vi "OP600ZP_FDT_FIN.vi"(8 "errin":errorcluster) -> (0 "errout":errorcluster caption="sortie d'erreur", 1 "ToBDD":T1, 2 "Log":string, 3 "is OK?":bool)   [LabVIEW 2020]
uses:
  OP600ZP_VGConf.vi
  VG/IS30%.vi
panel:
  out "PASS/FAIL?":string
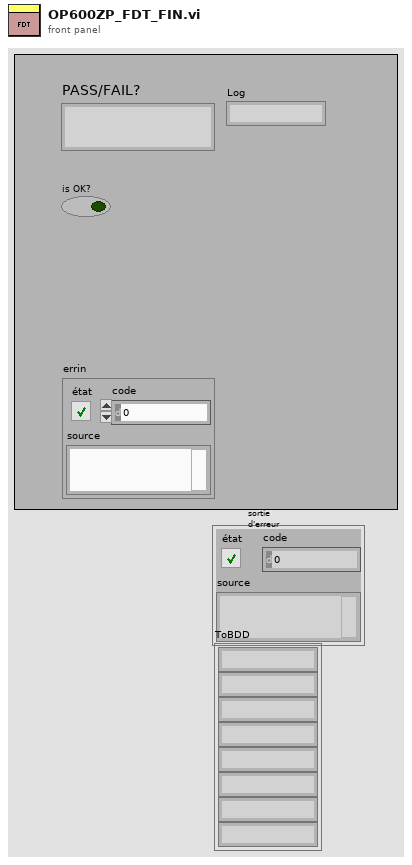
[diagram p1: front panel]
types:
  T1 = cluster{string, string, string, string, string, string, string, string}
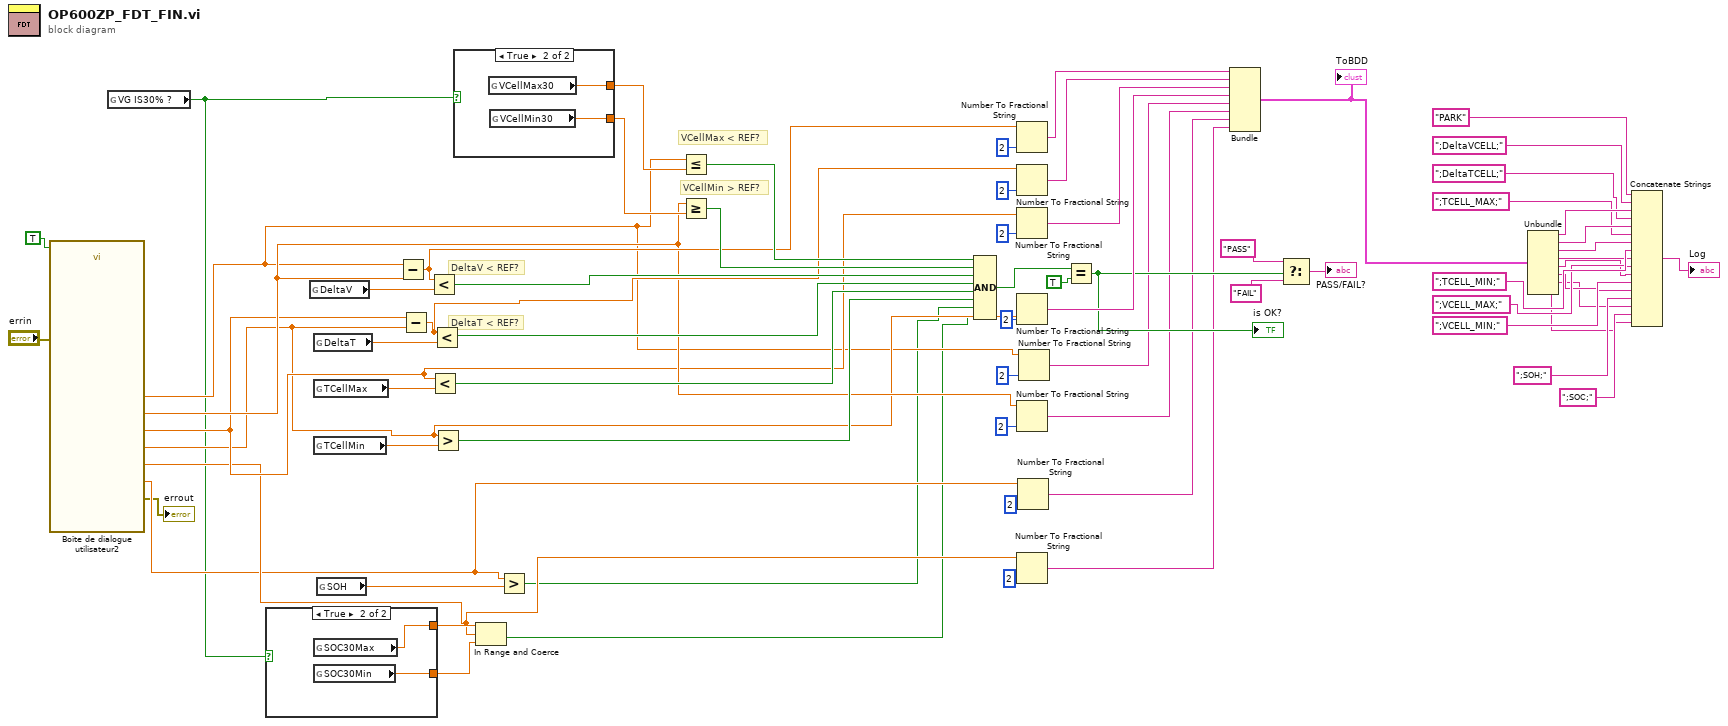
[diagram p0: block diagram]
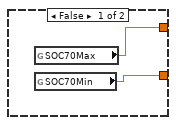
[diagram p2: hidden frame]
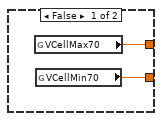
[diagram p3: hidden frame]
diagram:
  # "DeltaT < REF?"
  # "DeltaV < REF?"
  # "VCellMin > REF?"
  # "VCellMax < REF?"
  n1 = call "Boîte de dialogue utilisateur2"("Enable"=TRUE, "error in (no error)"="errin") -> ("SOH"=w11:dbl, "SOC"=w25:dbl, "Min Cell Temperature"=w29:dbl, "Max Cell Temperature"=w30:dbl, "Min Cell Voltage"=w36:dbl, "Max Cell Voltage"=w26:dbl, "error out"=→"errout":errorcluster)  [unwired: 9 in, 2 out]
  n2 = global read "IS30%.vi" "VG IS30% ?"() -> (w4:bool)
  n3 = case shown="True" w4 {
    tunnel: [w72 w74] -> w34
    tunnel: [w71 w73] -> w33
    frame False {
      n4 = global read "OP600ZP_VGConf.vi" "SOC70Max"() -> (w72:dbl)
      n5 = global read "OP600ZP_VGConf.vi" "SOC70Min"() -> (w71:dbl)
    }
    frame True {
      n6 = global read "OP600ZP_VGConf.vi" "SOC30Max"() -> (w74:dbl)
      n7 = global read "OP600ZP_VGConf.vi" "SOC30Min"() -> (w73:dbl)
    }
  }
  n8 = global read "OP600ZP_VGConf.vi" "DeltaV"() -> (w60:dbl)
  n9 = global read "OP600ZP_VGConf.vi" "DeltaT"() -> (w59:dbl)
  n10 = global read "OP600ZP_VGConf.vi" "TCellMax"() -> (w53:dbl)
  n11 = global read "OP600ZP_VGConf.vi" "TCellMin"() -> (w54:dbl)
  n12 = global read "OP600ZP_VGConf.vi" "SOH"() -> (w32:dbl)
  n13 = Subtract(x=w26, y=w36) -> (x-y=w50:dbl)
  n14 = Subtract(x=w30, y=w29) -> (x-y=w49:dbl)
  n15 = Less?(x=w50, y=w60) -> (x < y?=w57:bool)
  n16 = Less?(x=w30, y=w53) -> (x < y?=w52:bool)
  n17 = Less?(x=w49, y=w59) -> (x < y?=w58:bool)
  n18 = Greater?(x=w29, y=w54) -> (0:w51:bool)
  n19 = case shown="True" w4 {
    tunnel: [w76 w78] -> w28
    tunnel: [w75 w77] -> w48
    frame False {
      n20 = global read "OP600ZP_VGConf.vi" "VCellMax70"() -> (w76:dbl)
      n21 = global read "OP600ZP_VGConf.vi" "VCellMin70"() -> (w75:dbl)
    }
    frame True {
      n22 = global read "OP600ZP_VGConf.vi" "VCellMax30"() -> (w78:dbl)
      n23 = global read "OP600ZP_VGConf.vi" "VCellMin30"() -> (w77:dbl)
    }
  }
  n24 = In Range and Coerce(upper limit=w34, x=w25, lower limit=w33) -> (In Range?=w2:bool)  [unwired: 1 out]
  n25 = Greater?(x=w11, y=w32) -> (0:w3:bool)
  n26 = Less Or Equal?(x=w26, y=w28) -> (x <= y?=w55:bool)
  n27 = Greater Or Equal?(x=w36, y=w48) -> (x >= y?=w56:bool)
  n28 = Compound Arithmetic op=AND ("Opérateur arithmétique")(w55, w56, w57, w58, w52, w51, w3, w2) -> (w66:bool)
  n29 = Number To Fractional String(number=w50, precision (6)=i16 2 ("précision (6)")) -> (F-format string=w70:string)  [unwired: 2 in]
  n30 = Number To Fractional String(number=w49, precision (6)=i16 2 ("précision (6)")) -> (F-format string=w69:string)  [unwired: 2 in]
  n31 = Number To Fractional String(number=w30, precision (6)=i16 2 ("précision (6)")) -> (F-format string=w68:string)  [unwired: 2 in]
  n32 = Number To Fractional String(number=w29, precision (6)=i16 2 ("précision (6)")) -> (F-format string=w67:string)  [unwired: 2 in]
  n33 = Number To Fractional String(number=w36, precision (6)=i16 2 ("précision (6)")) -> (F-format string=w47:string)  [unwired: 2 in]
  n34 = Number To Fractional String(number=w25, precision (6)=i16 2 ("précision (6)")) -> (F-format string=w10:string)  [unwired: 2 in]
  n35 = Number To Fractional String(number=w11, precision (6)=i16 2 ("précision (6)")) -> (F-format string=w9:string)  [unwired: 2 in]
  n36 = Number To Fractional String(number=w26, precision (6)=i16 2 ("précision (6)")) -> (F-format string=w27:string)  [unwired: 2 in]
  n37 = Equal?(x=w66, y=TRUE) -> (x = y?=w62:bool)
  "is OK?" <- w62
  n38 = Bundle(w70, w69, w68, w67, w27, w47, w9, w10) -> (w39:T1)  [unwired: 1 in]
  "ToBDD" <- w39
  n39 = Select ("Sélectionner")(t="PASS", s=w62, f="FAIL") -> (s? t:f=→"PASS/FAIL?":string)
  n40 = Unbundle(w39) -> (w23:string, w21:string, w19:string, w17:string, w15:string, w13:string, w7:string, w5:string)
  n41 = Concatenate Strings("PARK", ";DeltaVCELL;", w23, ";DeltaTCELL;", w21, ";TCELL_MAX;", w19, ";TCELL_MIN;", w17, ";VCELL_MAX;", w15, ";VCELL_MIN;", w13, ";SOH;" ("chaîne"), w7, ";SOC;" ("chaîne"), w5) -> (→"Log":string)
